vi "RF_Synth_commands.vi"(1 "Value":dbl, 2 "Parameter":T1(ring)) -> (0 "Command":string)   [LabVIEW 2013]
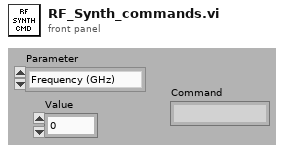
[diagram p1: front panel]
types:
  T1 = enum16{"Frequency (GHz)", "Power (dBm)", "Phase (deg)", "Output on?", "Trigger mode", "Set channel", "Init"}
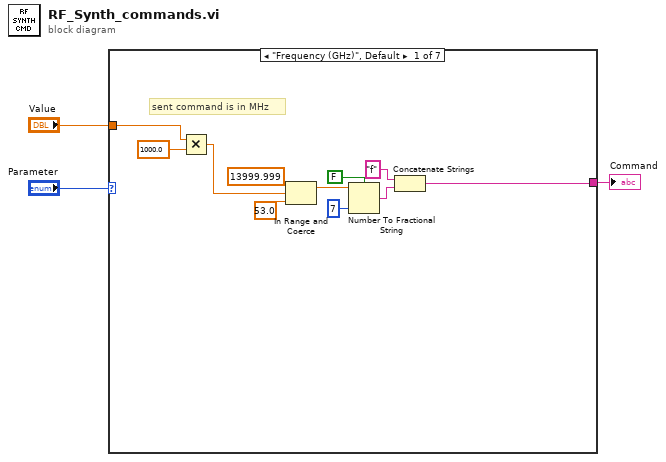
[diagram p0: block diagram]
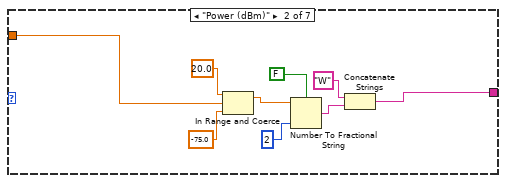
[diagram p2: hidden frame]
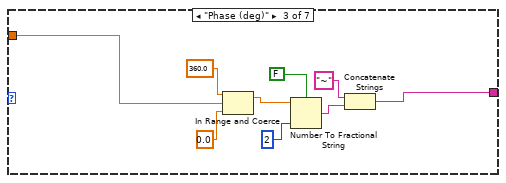
[diagram p3: hidden frame]
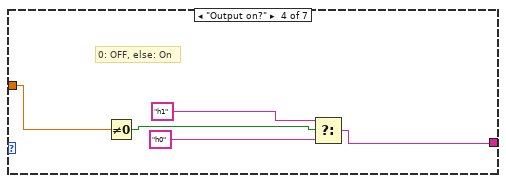
[diagram p4: hidden frame]
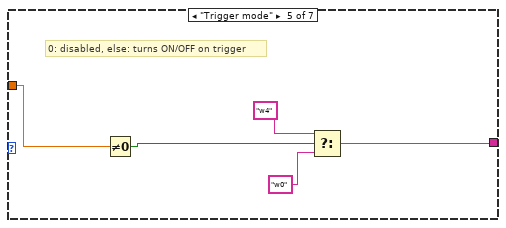
[diagram p5: hidden frame]
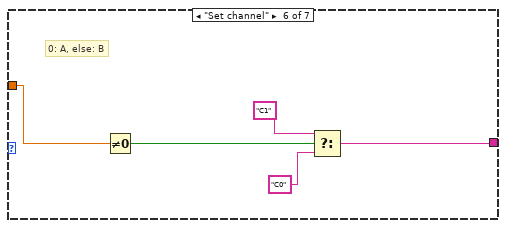
[diagram p6: hidden frame]
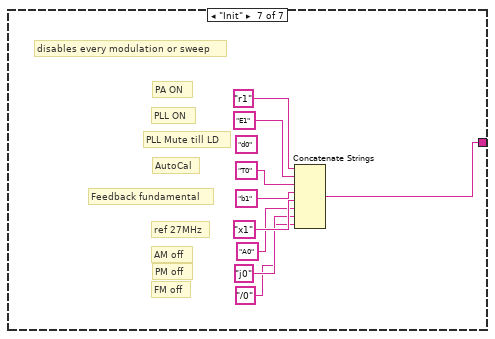
[diagram p7: hidden frame]
diagram:
  n1 = case shown="\"Frequency (GHz)\", Default" "Parameter" {
    tunnel: "Value" -> [w5 w15 w24 w35 w38 w43 _]
    tunnel: [w7 w16 w25 w33 w39 w44 w56] -> w2
    frame "Frequency (GHz)", Default {
      # "sent command is in MHz"
      n2 = Multiply(x=w5, y=1000.0) -> (x*y=w4:dbl)
      n3 = In Range and Coerce(upper limit=13999.999, x=w4, lower limit=53.0) -> (coerced(x)=w10:dbl)  [unwired: 1 out]
      n4 = Number To Fractional String(use system decimal point (T)=FALSE, number=w10, precision (6)=i16 7) -> (F-format string=w9:string)  [unwired: 1 in]
      n5 = Concatenate Strings("f" ("element"), w9) -> (w7:string)
    }
    frame "Power (dBm)" {
      n6 = In Range and Coerce(upper limit=20.0, x=w15, lower limit=-75.0) -> (coerced(x)=w21:dbl)  [unwired: 1 out]
      n7 = Number To Fractional String(use system decimal point (T)=FALSE, number=w21, precision (6)=i16 2) -> (F-format string=w19:string)  [unwired: 1 in]
      n8 = Concatenate Strings("W" ("string"), w19) -> (w16:string)
    }
    frame "Phase (deg)" {
      n9 = In Range and Coerce(upper limit=360.0, x=w24, lower limit=0.0) -> (coerced(x)=w30:dbl)  [unwired: 1 out]
      n10 = Number To Fractional String(use system decimal point (T)=FALSE, number=w30, precision (6)=i16 2) -> (F-format string=w28:string)  [unwired: 1 in]
      n11 = Concatenate Strings("~" ("string"), w28) -> (w25:string)
    }
    frame "Output on?" {
      # "0: OFF, else: On"
      n12 = Not Equal To 0?(x=w35) -> (x != 0?=w34:bool)
      n13 = Select(t="h1", s=w34, f="h0") -> (s? t:f=w33:string)
    }
    frame "Trigger mode" {
      # "0: disabled, else: turns ON/OFF on trigger"
      n14 = Not Equal To 0?(x=w38) -> (x != 0?=w40:bool)
      n15 = Select(t="w4", s=w40, f="w0") -> (s? t:f=w39:string)
    }
    frame "Set channel" {
      # "0: A, else: B"
      n16 = Not Equal To 0?(x=w43) -> (x != 0?=w45:bool)
      n17 = Select(t="C1", s=w45, f="C0") -> (s? t:f=w44:string)
    }
    frame "Init" {
      (unwired) "d0"
      # "AutoCal"
      # "Feedback fundamental"
      # "PLL Mute till LD"
      # "FM off"
      # "PM off"
      # "AM off"
      # "ref 27MHz"
      # "PLL ON"
      # "PA ON"
      # "disables every modulation or sweep"
      n18 = Concatenate Strings("r1", "E1", "T0", "b1", "x1", "A0", "j0", "/0") -> (w56:string)
    }
  }
  "Command" <- w2
